vi "Queue Driver.vi"(0 "Cases":string[](array[string]), 2 "Queue Name":string, 11 "Error In":errorcluster, 13 "Operation":T1=enum."Enqueue") -> (4 "Dequeued Case":string, 15 "Error Out":errorcluster)   [LabVIEW 2019, in "Car Wash.lvlib"]
doc: "This VI is used as a queue driver. It stores the queue reference and performs the below functions\nCreate Q\nEnqueue 1 elements\nEnqueue N elements\nEnstack 1 elements\nDequeue\nFlush Q\nDestroy Q"
uses:
  Car Wash.lvlib
  Controls/Queue Operations.ctl
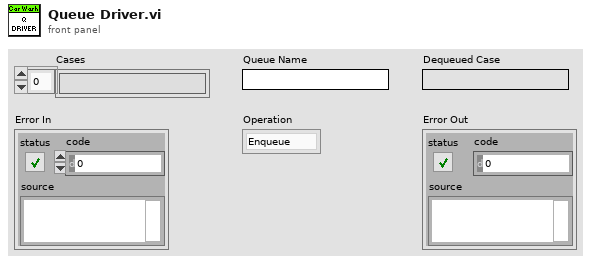
[diagram p1: front panel]
types:
  T1 = typedef "Car Wash.lvlib/Queue Operations.ctl" = enum16{"Create", "Enqueue", "Enstack", "Dequeue", "Flush", "Release"}
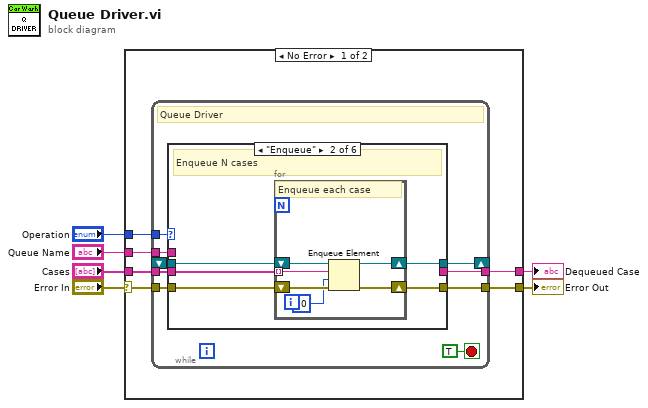
[diagram p0: block diagram]
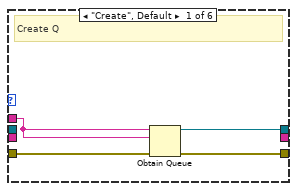
[diagram p2: hidden frame]
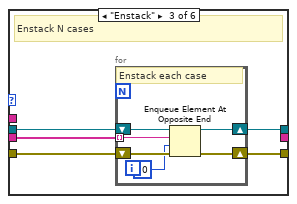
[diagram p3: hidden frame]
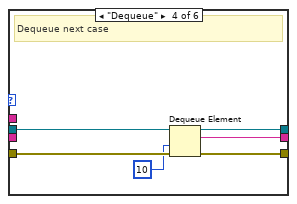
[diagram p4: hidden frame]
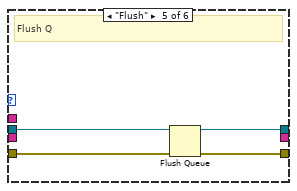
[diagram p5: hidden frame]
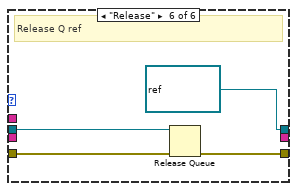
[diagram p6: hidden frame]
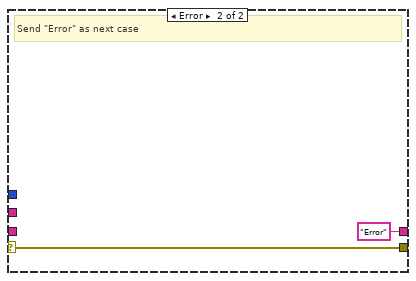
[diagram p7: hidden frame]
diagram:
  n1 = case shown="No Error" "Error In" {
    selector: "Error In" -> [w12 w63]
    tunnel: "Operation" -> [w11 _]
    tunnel: "Cases" -> [w10 _]
    tunnel: [w9 w63] -> w3
    tunnel: [w8 "Error"] -> w2
    tunnel: "Queue Name" -> [w7 _]
    frame No Error {
      n2 = while {
        tunnel: w12 -> [w19]
        tunnel: w11 -> [w21]
        tunnel: w10 -> [w20]
        tunnel: [w18] -> w9
        shift-right: [w16] -> _
        shift-left: _ -> [w17]
        tunnel: [w15] -> w8
        tunnel: w7 -> [w13]
        stop <- TRUE stop-if-true
        # "Queue Driver"
        n3 = case shown="\"Enqueue\"" w21 {
          tunnel: w20 -> [_ w28 w39 _ _ _]
          tunnel: w19 -> [w25 w30 w41 w50 w54 w59]
          tunnel: [w24 w29 w40 w53 w57 w61] -> w18
          tunnel: [w23 w26 w37 w52 w56 refnum<queue> refnum ("queue out")] -> w16
          tunnel: w17 -> [_ w27 w38 w51 w55 w60]
          tunnel: [_ _ _ w48 _ _] -> w15
          tunnel: w13 -> [w22 _ _ _ _ _]
          frame "Create", Default {
            # "Create Q"
            n4 = Obtain Queue(name (unnamed)=w22, element data type=w22, error in (no error)=w25) -> (queue out=w23:refnum<queue>, error out=w24:errorcluster)  [unwired: 2 in, 1 out]
          }
          frame "Enqueue" {
            # "Enqueue N cases"
            n5 = for {
              shift-right: [w35] -> w29
              shift-left: w30 -> [w36]
              tunnel: w28 -> [w34] mode=indexing
              shift-right: [w32] -> w26
              shift-left: w27 -> [w31]
              # "Enqueue each case"
              n6 = Enqueue Element(queue=w31, element=w34, timeout in ms (-1)=10, error in (no error)=w36) -> (queue out=w32:refnum<queue>, error out=w35:errorcluster)  [unwired: 1 out]
            }
          }
          frame "Enstack" {
            # "Enstack N cases"
            n7 = for {
              shift-right: [w46] -> w40
              shift-left: w41 -> [w47]
              tunnel: w39 -> [w45] mode=indexing
              shift-right: [w43] -> w37
              shift-left: w38 -> [w44]
              # "Enstack each case"
              n8 = Enqueue Element At Opposite End(queue=w44, element=w45, timeout in ms (-1)=10, error in (no error)=w47) -> (queue out=w43:refnum<queue>, error out=w46:errorcluster)  [unwired: 1 out]
            }
          }
          frame "Dequeue" {
            # "Dequeue next case"
            n9 = Dequeue Element(queue=w51, timeout in ms (-1)=10, error in (no error)=w50) -> (queue out=w52:refnum<queue>, element=w48:string, error out=w53:errorcluster)  [unwired: 1 out]
          }
          frame "Flush" {
            # "Flush Q"
            n10 = Flush Queue(queue=w55, error in (no error)=w54) -> (queue out=w56:refnum<queue>, error out=w57:errorcluster)  [unwired: 1 out]
          }
          frame "Release" {
            # "Release Q ref"
            n11 = Release Queue(queue=w60, error in (no error)=w59) -> (error out=w61:errorcluster)  [unwired: 1 in, 2 out]
          }
        }
      }
    }
    frame Error {
      # "Send \"Error\" as next case"
    }
  }
  "Error Out" <- w3
  "Dequeued Case" <- w2
